vi "Find SC.vi"(8 "error in (no error)":errorcluster, 11 "UV-VIS in":refnum<class "UV-VIS.lvclass">) -> (0 "error out":errorcluster, 3 "UV-VIS out":refnum<class "UV-VIS.lvclass">)   [LabVIEW 2015, in "UV-VIS.lvclass"]
uses:
  UV-VIS.lvclass
panel:
  out "in":dbl[](graph) caption="Data Values"
  out "out":dbl[](graph) caption="Data Values"
  out "position":i32
  out "II channel out":i32[][](array[numeric])
  out "I channel out":i32[][](array[numeric])
  in  "II channel":i32[][](array[numeric])
  in  "I channel":i32[][](array[numeric])
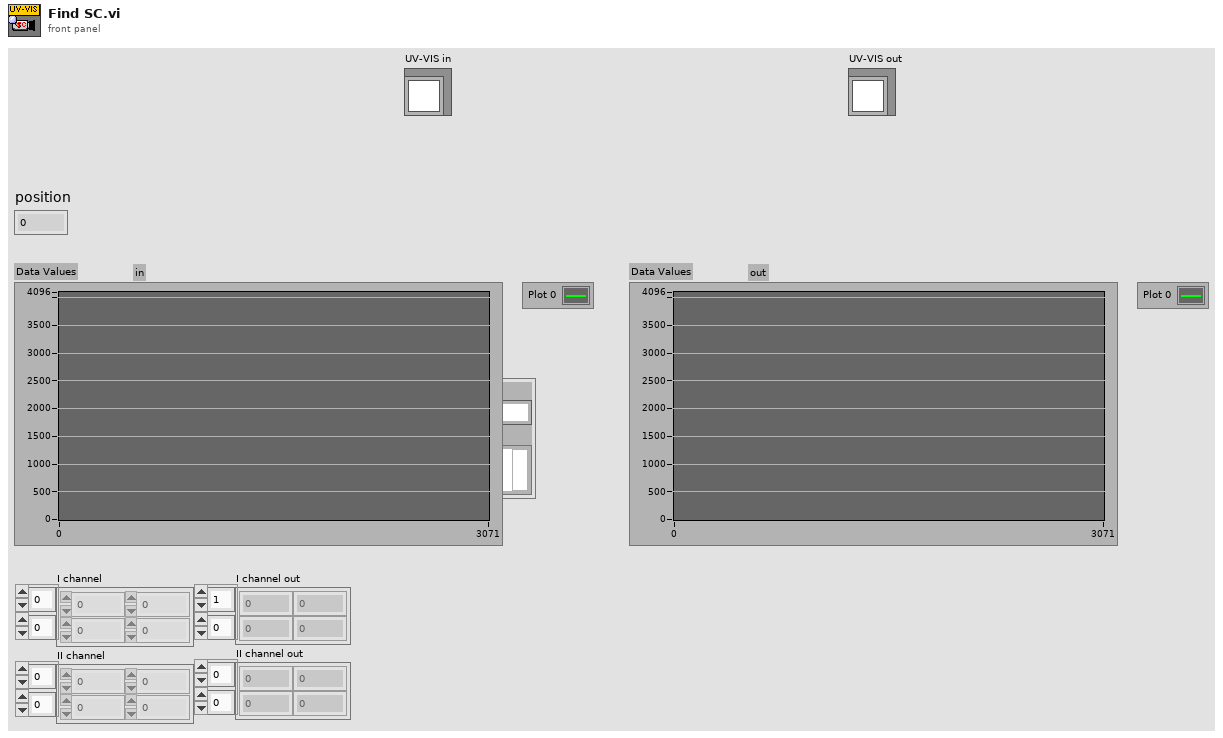
[diagram p1: front panel]
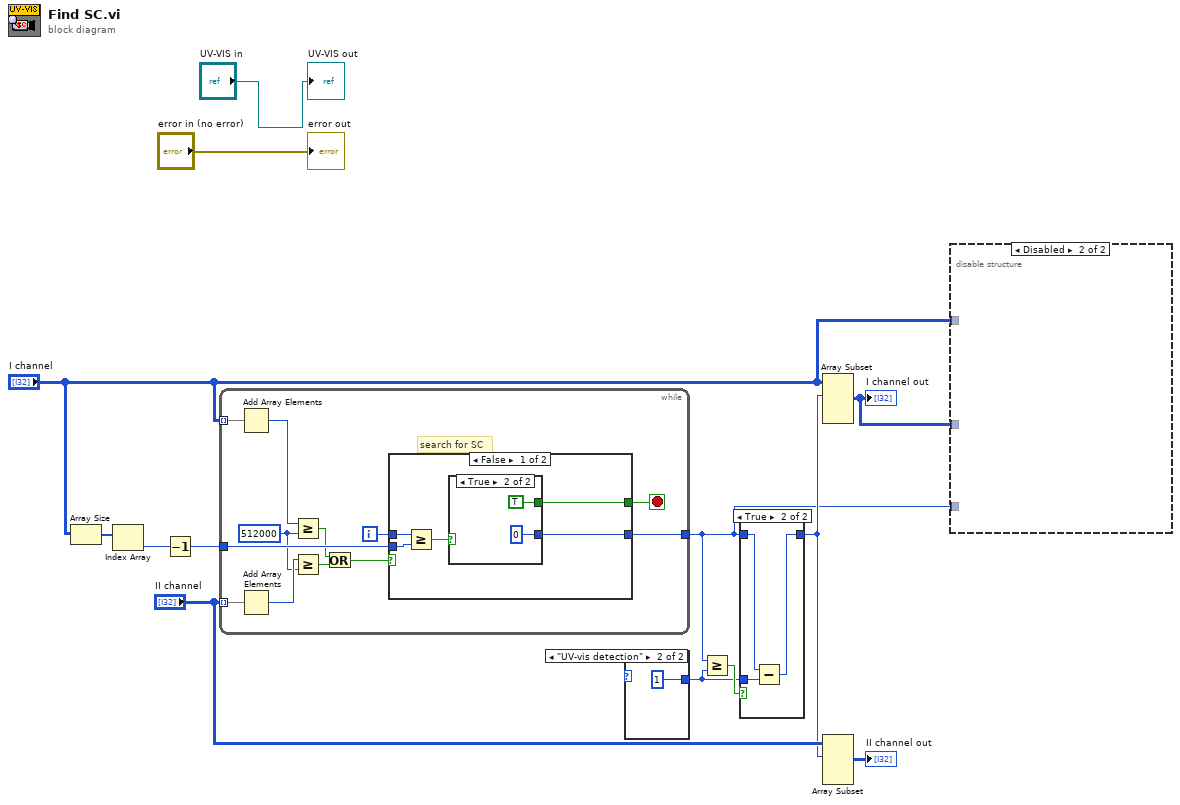
[diagram p0: block diagram]
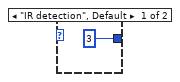
[diagram p2: hidden frame]
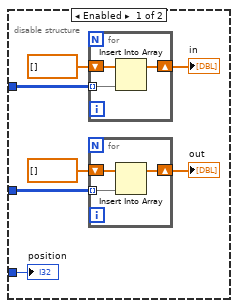
[diagram p4: hidden frame]
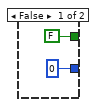
[diagram p5: hidden frame]
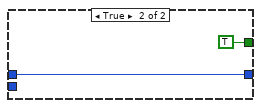
[diagram p6: hidden frame]
diagram:
  n1 = Array Size(array="I channel") -> (size(s)=w8:i32[])
  n2 = Index Array(array=w8) -> (element=w4:i32)  [unwired: 1 in]
  n3 = Decrement(x=w4) -> (x-1=w3:i32)
  n4 = while {
    tunnel: "I channel" -> [w21] mode=indexing
    tunnel: "II channel" -> [w20] mode=indexing
    tunnel: [w24] -> w7
    tunnel: w3 -> [w22]
    i -> [w23]
    stop <- w25 stop-if-true
    w17 = 512000 ("y")
    # "search for SC"
    n5 = Add Array Elements(numeric array=w21) -> (sum=w19:i32)
    n6 = Add Array Elements(numeric array=w20) -> (sum=w18:i32)
    n7 = Greater Or Equal?(x=w19, y=w17) -> (x >= y?=w16:bool)
    n8 = Greater Or Equal?(x=w18, y=w17) -> (x >= y?=w15:bool)
    n9 = Or(x=w16, y=w15) -> (x .or. y?=w14:bool)
    n10 = case shown="False" w14 {
      tunnel: [w27 TRUE] -> w25
      tunnel: [w28 w35] -> w24
      tunnel: w23 -> [w30 w35]
      tunnel: w22 -> [w26 _]
      frame False {
        n11 = Greater Or Equal?(x=w30, y=w26) -> (x >= y?=w29:bool)
        n12 = case shown="True" w29 {
          tunnel: [0 0] -> w28
          tunnel: [FALSE TRUE] -> w27
          frame False {
          }
          frame True {
          }
        }
      }
      frame True {
      }
    }
  }
  n13 = case shown="\"UV-vis detection\"" {
    selector: _ -> [_ _]
    tunnel: [3 ("y") 1 ("y")] -> w5
    frame "IR detection", Default {
    }
    frame "UV-vis detection" {
    }
  }
  n14 = Greater Or Equal?(x=w7, y=w5) -> (x >= y?=w11:bool)
  n15 = case shown="True" w11 {
    tunnel: [w39 w41] -> w10
    tunnel: w7 -> [w39 w42]
    tunnel: w5 -> [_ w40]
    frame False {
    }
    frame True {
      n16 = Subtract(x=w42, y=w40) -> (x-y=w41:i32)
    }
  }
  n17 = Array Subset(array="I channel", index (row)=w10) -> (w6:i32[][])  [unwired: 3 in]
  "I channel out" <- w6
  n18 = Array Subset(array="II channel", index (row)=w10) -> (→"II channel out":i32[][])  [unwired: 3 in]
  n19 = disable-structure shown="Disabled" {
    disable-tunnel: "I channel" -> [w47 _]
    disable-tunnel: w6 -> [w44 _]
    disable-tunnel: w7 -> [w43 _]
    frame Enabled {
      n20 = for {
        tunnel: w47 -> [w53] mode=indexing
        shift-right: [w54] -> w48
        shift-left: dbl[] [] ("tableau") -> [w55]
        n21 = Insert Into Array(array=w55, new element=w53) -> (w54:dbl[])  [unwired: 1 in]
      }
      "in" <- w48
      n22 = for {
        tunnel: w44 -> [w50] mode=indexing
        shift-right: [w51] -> w46
        shift-left: dbl[] [] ("tableau") -> [w52]
        n23 = Insert Into Array(array=w52, new element=w50) -> (w51:dbl[])  [unwired: 1 in]
      }
      "out" <- w46
      "position" <- w43
    }
    frame Disabled {
    }
  }
  "error out" <- "error in (no error)"
  "UV-VIS out" <- "UV-VIS in"
